vi "Auto Home.vi"(7 "Arm ID":i32(ring)=1 items=["Left Arm", "Right Arm"], 10 "ToolInsertionOffset":dbl=-54.76, 11 "ToolType":i32=6) -> ()   [LabVIEW 2016]
uses:
  <vilib>/Platform/TimedLoop/XDataNode/timing_clust.ctl
  <vilib>/Platform/TimedLoop/XDataNode/nitl_modes.ctl
  <vilib>/Platform/TimedLoop/XDataNode/wakeup.ctl
  Subsystems/Global Variables.vi
  <vilib>/platform/TimedLoop/XDataNode/XDataNode.xnode
  <vilib>/Platform/TimedLoop/XDataNode/XDNodeRunTimeDep.lvlib
panel:
  out "Homing Status":bool[](array[boolean])
  in  "Set Tool Type":bool
  in  "Homing XYZ Stage":bool
  in  "Homing Tool":bool
  in  "Homing Arm":bool
  # "Tool Configuration Commands"
  # "Homing Commands"
  # "Home Arm Done"
  # "Home Tool Done"
  # "Home XYZ Stage Done"
  # "For debug only, No need to use this button during labview operation, if does, then the low level control will be terminated, and everything will have to be rerestarted including homing"
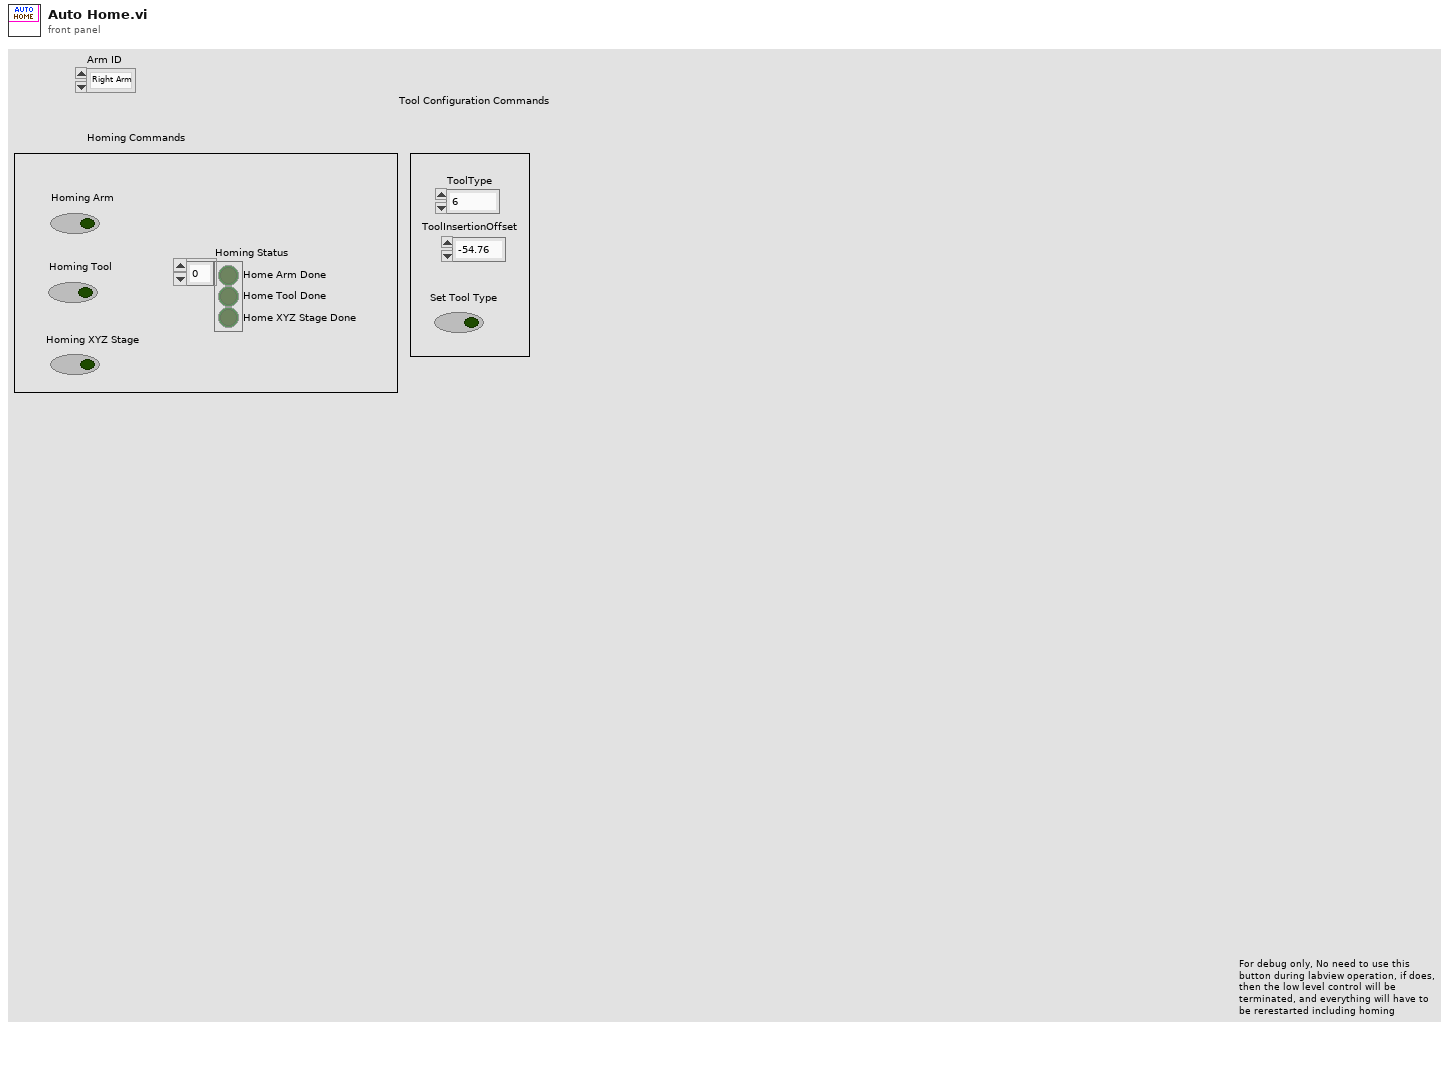
[diagram p1: front panel]
types:
  T1 = typedef "XDNodeRunTimeDep.lvlib/timing_clust.ctl" = cluster{"Expected End [f-1]":u64, "Actual End [f-1]":u64, "Finished Late? [f-1]":bool, "Expected End [i-1]":u64, "Actual End [i-1]":u64, "Finished Late? [i-1]":bool, "Expected Start [i]":u64, "Actual Start [i]":u64, "Expected Start [f]":u64, "Actual Start [f]":u64, "Source Name":string, "Structure Name":string, "Period":i64, "Deadline":i64, "Offset":i64, "Start":i64, "Priority":i32, "Timeout":i32, "Mode":T2, "Wakeup Reason":T3, "Error":errorcluster, "Source Type":string, "Secondary Source Type":string, "Global End Time":u64, "Global Start Time":u64, "Frame Duration":u64, "Iteration Duration":u64, "Assigned CPU":i32, "I/O Scan Engine Mode":u32}
  T2 = typedef "XDNodeRunTimeDep.lvlib/nitl_modes.ctl" = enum32{"No Change", "Process missed periods, maintain original phase", "Discard missed periods, maintain original phase", "Process missed periods, ignore original phase", "Discard missed periods, ignore original phase"}
  T3 = typedef "XDNodeRunTimeDep.lvlib/wakeup.ctl" = enum32{"Normal", "Aborted", "Asynchronous wakeup", "Timing source error", "Timed loop error", "Timeout"}
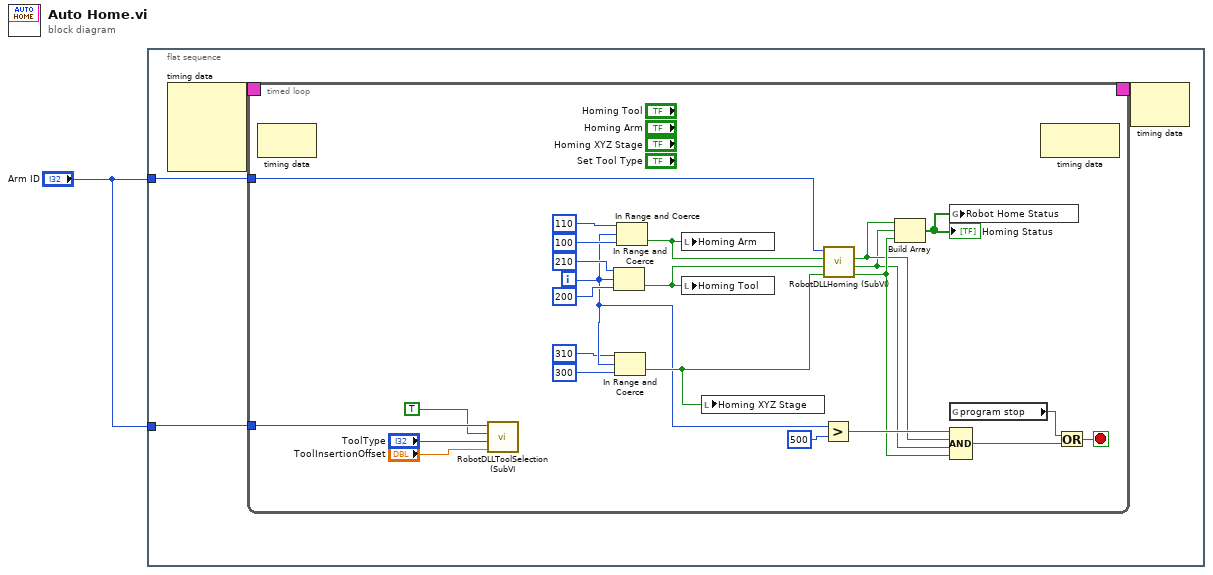
[diagram p0: block diagram]
diagram:
  n1 = flat-sequence {
    tunnel: "Arm ID" -> [w5]
    tunnel: "Arm ID" -> [w2]
    frame #0 {
      n2 = node-c288() -> (w4:T1)  [unwired: 4 in]
      n3 = timed-loop {
        timing: w4 -> [_]
        timing-out: [_] -> w3
        tunnel: w5 -> [w11]
        tunnel: w2 -> [w29]
        i -> [w10]
        stop <- w21 stop-if-true
        n4 = node-c288() -> ()  [unwired: 1 in, 1 out]
        n5 = call "RobotDLLToolSelection (SubVI.vi"("tool insertion offset"="ToolInsertionOffset", "ToolType"="ToolType", "Set Tool Type"=TRUE, "ArmID"=w29) -> ()  [unwired: 4 in]
        n6 = In Range and Coerce(upper limit=210, x=w10, lower limit=200) -> (In Range?=w19:bool)  [unwired: 1 out]
        n7 = In Range and Coerce(upper limit=310, x=w10, lower limit=300) -> (In Range?=w13:bool)  [unwired: 1 out]
        n8 = In Range and Coerce(upper limit=110, x=w10, lower limit=100) -> (In Range?=w15:bool)  [unwired: 1 out]
        n9 = local write "Homing Arm"(w15) -> ()
        n10 = local write "Homing Tool"(w19) -> ()
        n11 = local write "Homing XYZ Stage"(w13) -> ()
        n12 = Greater?(x=w10, y=500) -> (0:w23:bool)
        n13 = call "RobotDLLHoming (SubVI).vi"("Homing XYZ Stage"=w13, "Homing Tool"=w19, "Homing Arm"=w15, "ArmID"=w11) -> ("Homing XYZ Stage Done"=w12:bool, "Homing Tool Done"=w8:bool, "Homing Arm Done"=w9:bool)  [unwired: 1 in]
        n14 = Build Array(w9, w8, w12) -> (w18:bool[])
        "Homing Status" <- w18
        n15 = global write "Global Variables.vi" "Robot Home Status"(w18) -> ()
        n16 = global read "Global Variables.vi" "program stop"() -> (w20:bool)
        n17 = Compound Arithmetic op=AND(w23, w9, w8, w12) -> (w22:bool)
        n18 = node-c288() -> ()  [unwired: 1 in, 1 out]
        n19 = Or(x=w20, y=w22) -> (x .or. y?=w21:bool)
      }
      n20 = node-c288(w3) -> ()  [unwired: 1 out]
    }
  }
